vi "Unregister.vi"(8 "error in":errorcluster, 11 "Message Waiter in":refnum<class "Message Waiter.lvclass">) -> (0 "error out":errorcluster, 3 "Message Waiter out":refnum<class "Message Waiter.lvclass">)   [LabVIEW 2018, in "PCANBasic.lvlib" / "Message Waiter.lvclass"]
uses:
  Message Waiter.lvclass
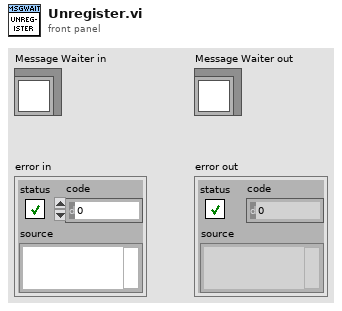
[diagram p1: front panel]
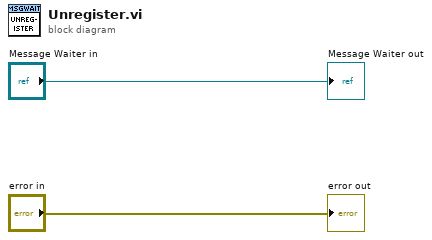
[diagram p0: block diagram]
diagram:
  "error out" <- "error in"
  "Message Waiter out" <- "Message Waiter in"
